vi "CollectorWrap.vi"(7 "Action":T1) -> ()   [LabVIEW 2013]
uses:
  Autonomous/DoubleSolenoidControl.ctl
  Autonomous/RollerStates.ctl
  CollectorWrapAction.ctl
panel:
  out "error out":errorcluster
  in  "error in":errorcluster
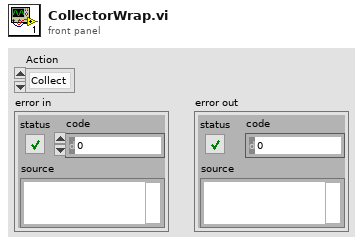
[diagram p1: front panel]
types:
  T1 = typedef "CollectorWrapAction.ctl" = enum16{"Collect", "Stop"}
  T2 = typedef "RollerStates.ctl" = enum16{"Init", "Off", "Forward", "Reverse"}
  T3 = typedef "DoubleSolenoidControl.ctl" = enum16{"Init", "Out", "In", "Middle"}
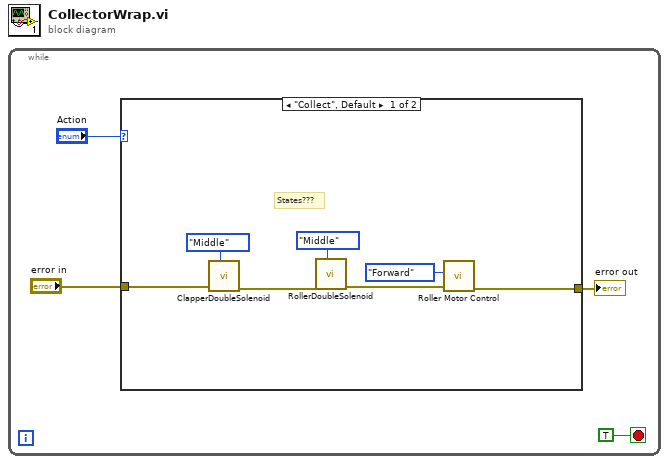
[diagram p0: block diagram]
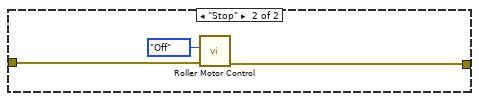
[diagram p2: hidden frame]
diagram:
  n1 = while {
    stop <- TRUE stop-if-true
    n2 = case shown="\"Collect\", Default" "Action" {
      tunnel: "error in" -> [w10 w14]
      tunnel: [w5 w13] -> w1
      frame "Collect", Default {
        # "States???"
        n3 = call "ClapperDoubleSolenoid.vi"("State"=DoubleSolenoidControl."Middle", "Error in"=w10) -> ("Error out"=w9:errorcluster)  [unwired: 9 in]
        n4 = call "RollerDoubleSolenoid.vi"("State"=DoubleSolenoidControl."Middle", "Error in"=w9) -> ("Error out"=w7:errorcluster)  [unwired: 9 in]
        n5 = call "Roller Motor Control.vi"("Error in"=w7, "RollerState"=RollerStates."Forward") -> ("Error out"=w5:errorcluster)  [unwired: 9 in]
      }
      frame "Stop" {
        n6 = call "Roller Motor Control.vi"("Error in"=w14, "RollerState"=RollerStates."Off") -> ("Error out"=w13:errorcluster)  [unwired: 9 in]
      }
    }
    "error out" <- w1
  }
